vi "Global 6KA.vi"() -> ()   [LabVIEW 2009]
panel:
  in  "Manual RMS wave":dbl[](array[numeric])
  in  "end time index":i32
  in  "start time index":i32
  in  "Refine current wave":dbl[](array[numeric])
  in  "DAQ speed":i16
  in  "Current Range":i16
  in  "current wave":dbl[][](array[numeric])
  in  "current":dbl
  in  "power on time":dbl
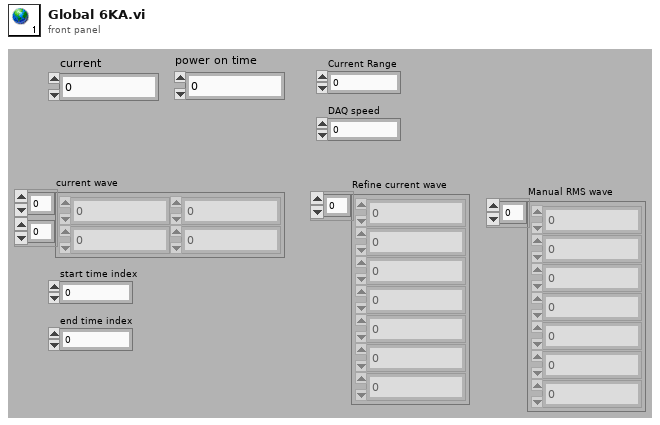
[diagram p1: front panel]
diagram:
